vi "TCP (Listener).vi"(10 "bytes to read":i32, 11 "port":u16) -> (2 "error out":errorcluster, 3 "data out":string)   [LabVIEW 2013]
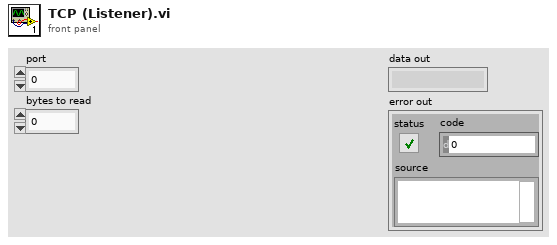
[diagram p1: front panel]
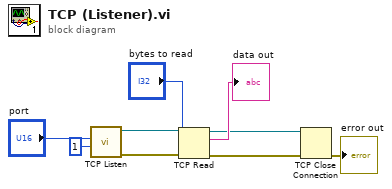
[diagram p0: block diagram]
diagram:
  n1 = call <vilib>:"TCP Listen.vi"("timeout ms (wait forever: -1)"=1, "port"="port") -> ("error out"=w6:errorcluster, "connection ID"=w7:refnum<k5>)  [unwired: 5 in, 3 out]
  n2 = TCP Read(connection ID=w7, bytes to read="bytes to read", error in (no error)=w6) -> (connection ID out=w4:refnum<k5>, data out=→"data out":string, error out=w3:errorcluster)  [unwired: 2 in]
  n3 = TCP Close Connection(connection ID=w4, error in (no error)=w3) -> (error out=→"error out":errorcluster)  [unwired: 1 in, 1 out]
